vi "Dashboard globals.vi"() -> ()   [LabVIEW 2018]
panel:
  in  "Right y":sgl
  in  "Left y":sgl
  in  "Right x":sgl
  in  "Left x":sgl
  in  "Right width":sgl
  in  "Left width":sgl
  in  "Right height":sgl
  in  "Left height":sgl
  out "Desired Target":T1(radio)=enum."Ship End - Left"
  in  "Enable Vision\nProcessing":bool
  # "Side of Ship"
  # "End of Ship"
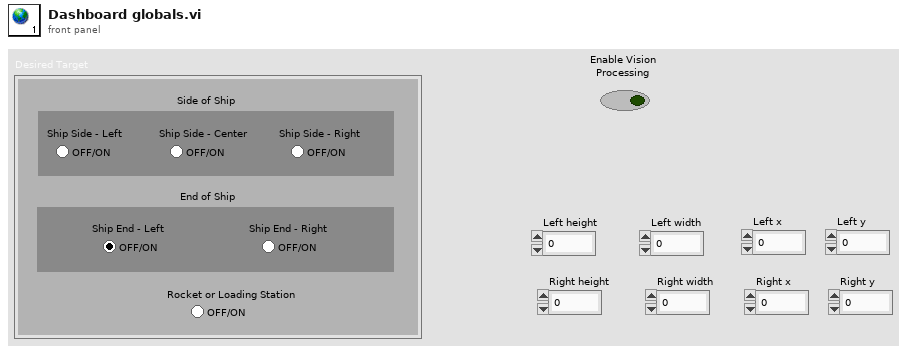
[diagram p1: front panel]
types:
  T1 = enum32{"Ship Side - Left", "Ship Side - Center", "Ship Side - Right", "Ship End - Left", "Ship End - Right", "Rocket or Loading Station"}
diagram:
